vi "KSB.vi"(0 "System no.":i32=1 min=1 max=4 step=1, 1 "Name":string, 2 "Axes to set":string[](array[string]), 3 "Position values":dbl[](array[numeric]) format="%.6f", 4 "No.of digits":i16=4, 5 "error in":errorcluster) -> (19 "error out":errorcluster)   [LabVIEW 2020]
doc: "Defines a base coordinate system (KSB-Type) and queries ERR?. Use KSB in order to change the orientation of the base coordinate system.\nKSB only can rotate the coordinate system by 0, 90, 180, 270, -90, -180, -270 degrees. If there is already a coordinate system with the same name, KSB will replace it if it is not used. Activating a KSB type coordinate system (KEN.vi) does not cause any motion, and POS?.vi will report new position values. If the hexapod is moving, the command can be applied. All pivot point coordinates (SPI.vi) will remain. SPI.vi is allowed when a KSB type coordinate system is active. For new or replaced KSB type coordinate systems, the parent coordinate system will be set to the currently active KSB coordinate system. When replacing a coordinate system of this type, the chain relations will not be changed if the coordinate system to replace is of the same type. For axes which are not given, the position values will be set to 0. Coordinate system settings are volatile but can be saved as power-on default with WPA.vi using the password \"SKS\". This command requires command level 1 (CCL.vi).\n\nC-887, F-206, M-8X0: Only for GCS syntax version = GCS 2.0 or higher (Check with CSV?.vi. If CSV?.vi is not supported, syntax version is GCS 1.0)."
panel:
  # "Defines a Base coordinate system (KSB-Type) and queries ERR?. Use KSB \nin order to change the orientation of the Base coordinate system."
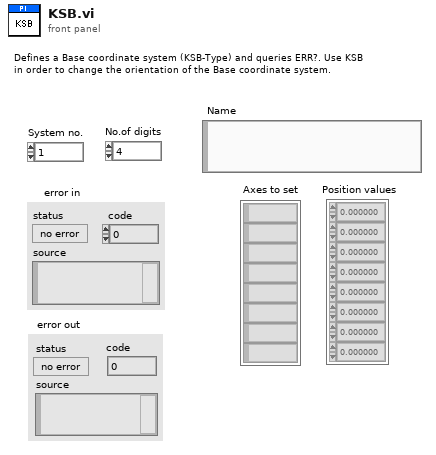
[diagram p1: front panel]
types:
  T1 = enum16{"Disable error check", "Force error check", "Use global settings"}
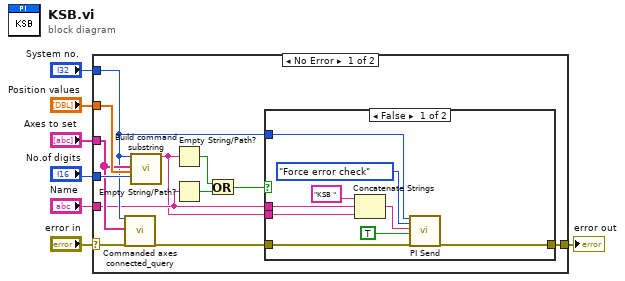
[diagram p0: block diagram]
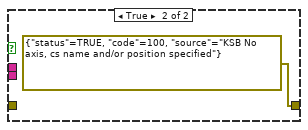
[diagram p2: hidden frame]
diagram:
  n1 = case shown="No Error" "error in" {
    selector: "error in" -> [w11 w30]
    tunnel: [w19 w30] -> w7
    tunnel: "Position values" -> [w18 _]
    tunnel: "No.of digits" -> [w17 _]
    tunnel: "System no." -> [w14 _]
    tunnel: "Axes to set" -> [w15 _]
    tunnel: "Name" -> [w13 _]
    frame No Error {
      n2 = call "Commanded axes connected_query.vi"("System no."=w14, "Commanded axes"=w15, "error in"=w11) -> ("error out"=w16:errorcluster)  [unwired: 1 in, 15 out]
      n3 = call "Build command substring.vi"("System no."=w14, "Affected axes"=w15, "Parameters"=w18, "No. of digits"=w17) -> ("Command substring"=w12:string)  [unwired: 3 in, 12 out]
      n4 = Empty String/Path?(string/path=w12) -> (empty?=w9:bool)
      n5 = Empty String/Path?(string/path=w13) -> (empty?=w10:bool)
      n6 = Or(x=w9, y=w10) -> (x .or. y?=w8:bool)
      n7 = case shown="False" w8 {
        tunnel: [w21 errorcluster {"status"=TRUE, "code"=100, "source"="KSB No axis, cs name and/or position specified"} ("error out")] -> w19
        tunnel: w12 -> [w28 _]
        tunnel: w16 -> [w27 _]
        tunnel: w14 -> [w22 _]
        tunnel: w13 -> [w23 _]
        frame False {
          n8 = Concatenate Strings("KSB ", w23, w28) -> (w25:string)
          n9 = call "PI Send.vi"("System no."=w22, "Error check settings"=T1."Force error check", "String to send"=w25, "Attach termination char.?"=TRUE ("Attach Linefeed?"), "error in"=w27) -> ("error out"=w21:errorcluster)  [unwired: 1 in, 13 out]
        }
        frame True {
        }
      }
    }
    frame Error {
    }
  }
  "error out" <- w7
